vi "Sub Initialize.vi"(8 "error in (no error)":errorcluster, 11 "Instrument Recorder in":refnum<class "RP Level.lvclass">) -> (0 "error out":errorcluster, 2 "Initialize Result":refnum<class "Acquired Result.lvclass">, 3 "Instrument Recorder out":refnum<class "RP Level.lvclass">)   [LabVIEW 2018, in "RP Level.lvclass"]
uses:
  RP Level.lvclass
  C:/github/2018/LabActor/Pulse Recorders/Pulse Recorder/Pulse Recorder.lvclass
  C:/github/2018/LabActor/Template Module/Template Module.lvclass
  NHMFL_Core/Libraries/Instruments/Results/Acquired Result/Acquired Result.lvclass
  NHMFL_Core/Libraries/Red Pitaya/Red Pitaya Digitizer/Red Pitaya Digitizer.lvclass
  C:/github/2018/NHMFL_Core/Libraries/Instruments/Pulse Driver/Pulse Driver.lvclass
  NHMFL_Core/Libraries/Red Pitaya/Red Pitaya Digitizer/Red Pitaya Digitizer.lvclass/Red Pitaya Digitizer.ctl
  Template Module/Template Module.lvclass/Template Module.ctl
  NHMFL_Core/Libraries/Red Pitaya/Red Pitaya Digitizer/Write Tigger level.vi
  Template Module/Write Configuration.vi
  Pulse Recorders/Pulse Recorder/Read Pulse driver.vi
  Pulse Recorders/Pulse Recorder/Write Pulse driver.vi
  NHMFL_Core/Libraries/Instruments/Pulse Driver/Pulse Driver.lvclass
  Pulse Recorders/Pulse Recorder/Pulse Recorder.lvclass
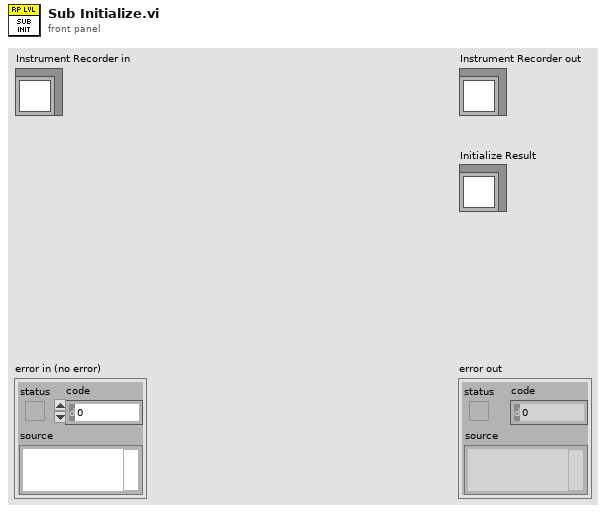
[diagram p1: front panel]
types:
  T1 = typedef "RP Level Configuration.ctl" = cluster{"Pre-trigger duration":dbl, "Post-trigger duration":dbl, "Rate":dbl, "Ranges":dbl[], "Re-name channels":string[], "Active channels":string, "External clock":bool, "Output delay":dbl, "Raising edge ":bool, "Trigger level":dbl}
  T2 = typedef "Pusle Driver Configuration.ctl" = cluster{"Pre-trigger duration":dbl, "Post-trigger duration":dbl, "Rate":dbl, "Ranges":dbl[], "Re-name channels":string[], "Active channels":string, "External clock":bool}
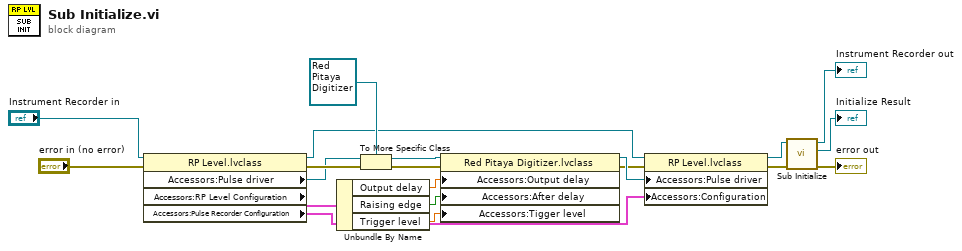
[diagram p0: block diagram]
diagram:
  n1 = property class="RP Level.lvclass"(reference="Instrument Recorder in", error in="error in (no error)") -> (reference out=w8:refnum<class "RP Level.lvclass">, error out=w17:errorcluster, "Accessors:Pulse driver"=w16:refnum<class "Pulse Driver.lvclass">, "Accessors:RP Level Configuration"=w13:T1, "Accessors:Pulse Recorder Configuration"=w3:T2)
  n2 = Unbundle By Name(w13) -> ("Output delay"=w12:dbl, "Raising edge"=w2:bool, "Trigger level"=w1:dbl)
  n3 = To More Specific Class(target class=refnum<class "Red Pitaya Digitizer.lvclass"> refnum ("Red Pitaya Digitizer.lvclass"), reference=w16, error in=w17) -> (specific class reference=w14:refnum<class "Red Pitaya Digitizer.lvclass">, error out=w11:errorcluster)
  n4 = property class="Red Pitaya Digitizer.lvclass"(reference=w14, error in=w11, "Accessors:Output delay"=w12, "Accessors:After delay"=w2, "Accessors:Tigger level"=w1) -> (reference out=w10:refnum<class "Red Pitaya Digitizer.lvclass">, error out=w7:errorcluster)
  n5 = property class="RP Level.lvclass"(reference=w8, error in=w7, "Accessors:Pulse driver"=w10, "Accessors:Configuration"=w3) -> (reference out=w4:refnum<class "RP Level.lvclass">, error out=w5:errorcluster)
  n6 = call-parent "Sub Initialize.vi"("error in (no error)"=w5, "Instrument Recorder in"=w4) -> ("error out"=→"error out":errorcluster, "Initialize Result"=→"Initialize Result":refnum<class "Acquired Result.lvclass">, "Instrument Recorder out"=→"Instrument Recorder out":refnum<class "RP Level.lvclass">)  [unwired: 7 in]
